vi "GenError.vi"(8 "error in (no error)":errorcluster, 10 "Code":i32) -> (0 "error out":errorcluster)   [LabVIEW 2015]
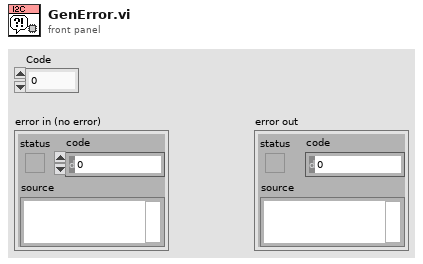
[diagram p1: front panel]
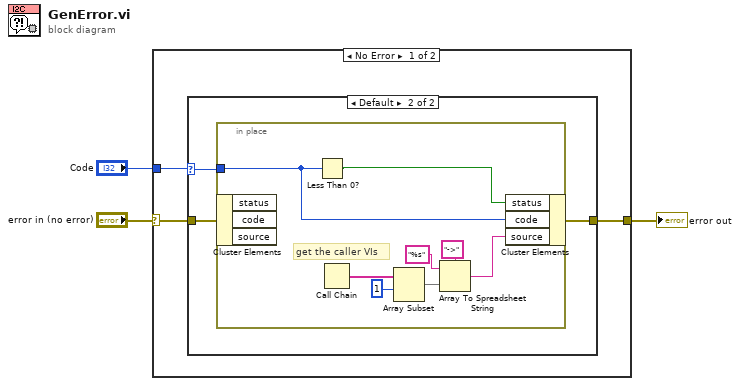
[diagram p0: block diagram]
diagram:
  n1 = case shown="No Error" "error in (no error)" {
    selector: "error in (no error)" -> [w6 w19]
    tunnel: [w5 w19] -> w3
    tunnel: "Code" -> [w4 _]
    frame No Error {
      n2 = case shown="Default" w4 {
        selector: w4 -> [_ w8]
        tunnel: w6 -> [w7 w10]
        tunnel: [w7 w9] -> w5
        frame 0 {
        }
        frame Default {
          n3 = in-place {
            in-place-border: w8 -> [w12]
            # "get the caller VIs"
            n4 = in-place-cluster #1(w10) -> ()  [unwired: 3 out]
            n5 = Less Than 0?(x=w12) -> (x < 0?=w11:bool)
            n6 = Call Chain() -> (call chain=w16:string[])
            n7 = Array Subset(array=w16, index=1 ("Array Index")) -> (w17:string[])  [unwired: 1 in]
            n8 = Array To Spreadsheet String(delimiter (Tab)="->", array=w17, 3:"%s" ("format string")) -> (spreadsheet string=w13:string)
            n9 = in-place-cluster #1("status"=w11, "code"=w12, "source"=w13) -> (w9:errorcluster)
          }
        }
      }
    }
    frame Error {
    }
  }
  "error out" <- w3
